vi "Close.vi"(8 "error in (no error)":errorcluster, 11 "VISA in":refnum<class "VISA.lvclass">) -> (0 "error out":errorcluster, 3 "VISA out":refnum<class "VISA.lvclass">)   [LabVIEW 2019, in "Protocols.lvlib" / "VISA.lvclass"]
uses:
  VISA.lvclass
  VISA.lvclass/VISA.ctl
  Read Ref.vi
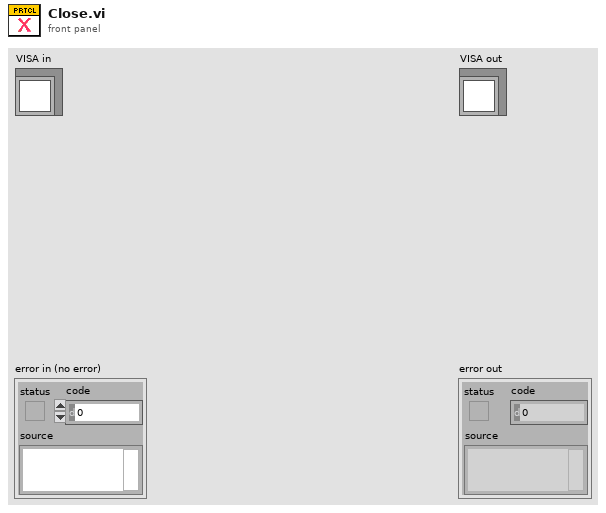
[diagram p1: front panel]
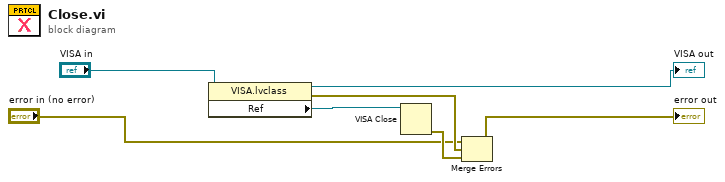
[diagram p0: block diagram]
diagram:
  n1 = property class="VISA.lvclass"(reference="VISA in") -> (reference out=→"VISA out":refnum<class "VISA.lvclass">, error out=w5:errorcluster, "Ref"=w7:refnum<visa-resource-name>)  [unwired: 1 in]
  n2 = VISA Close(VISA resource name=w7) -> (error out=w6:errorcluster)  [unwired: 1 in]
  n3 = Merge Errors("error in (no error)", w5, w6) -> (→"error out":errorcluster)
